vi "tm_getparameter_a.vi"(6 "Index":i32, 8 "error in (no error)":errorcluster, 10 "Parameter":u32(ring)=4215968 items=["SENSOR MODE"=4212128, "CCD MODE"=4212384, "READOUT MODE"=4211872, "ACTIVE VIEW INDEX"=4343136, "BITS PER CHANNEL"=4342976, "IMAGE PIXEL TYPE"=4343296, "BINNING"=4215968, "EXPOSURE TIME"=2049184, "CONTRAST GAIN"=3163312, "CONTRAST OFFSET"=3163328, "LIGHT MODE"=2114720, "SENSITIVITY"=2114992, "PHOTON IMAGING MODE"=2115200, "HIGH DYNAMIC RANGE MODE"=3163360, "WHITE BALANCE"=3163568, "TEMPERATURE"=2115232, "TEMPERATURE TARGET"=2115264, "SENSOR COOLER FAN"=2115296, "LINEBUNDLE HEIGHT"=4212192, "MECHANICAL SHUTTER"=2115488, "BACK FOCUS POSITION"=8422304, "TRIGGER CONNECTOR"=1066432, "TRIGGER SOURCE"=1066144, "OUTPUT TRIGGER SOURCE"=1852576, "TRIGGER GLOBAL EXPOSURE"=2049680, "FIRST TRIGGER BEHAVIOR"=2049696, "CHANNEL SYNC"=1852352, "READOUT DIRECTION"=4211904, "PRE HSYNC COUNT"=1852704, "INTERNAL LINE SPEED"=4191408, "INTERNAL LINE INTERVAL"=4191424], 11 "Handle in":u32) -> (0 "error out":errorcluster, 2 "Value out":dbl, 3 "Handle out":u32)   [LabVIEW 2015]
uses:
  tmcamcon.dll
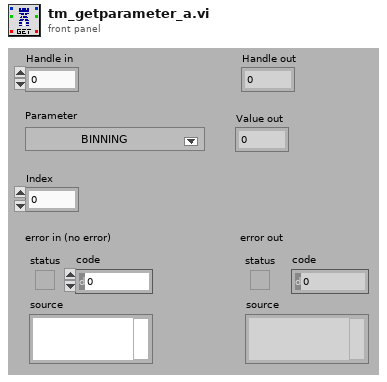
[diagram p1: front panel]
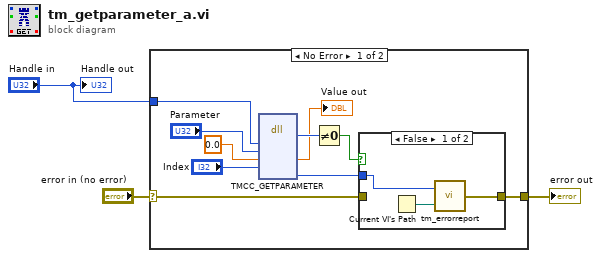
[diagram p0: block diagram]
diagram:
  n1 = case shown="No Error" "error in (no error)" {
    selector: "error in (no error)" -> [w8 w18]
    tunnel: [w5 w18] -> w2
    tunnel: "Handle in" -> [w12 _]
    frame No Error {
      n2 = dll-call lib="tmcamcon.dll" fn="TMCC_GETPARAMETER"("handle"=w12, "parameter"="Parameter", "value"=0.0, "view"="Index") -> ("return type"=w13:u32, "value"=→"Value out":dbl, "Erval"=w7:i32)  [unwired: 7 in, 2 out]
      n3 = Not Equal To 0?(x=w13) -> (x != 0?=w6:bool)
      n4 = case shown="False" w6 {
        tunnel: w8 -> [_ w17]
        tunnel: [w15 w17] -> w5
        tunnel: w7 -> [w14 _]
        frame False {
          n5 = Current VI's Path() -> (path=w16:path)
          n6 = call "tm_errorreport.vi"("Source"=w16, "Error"=w14) -> ("error out"=w15:errorcluster)
        }
        frame True {
        }
      }
    }
    frame Error {
    }
  }
  "error out" <- w2
  "Handle out" <- "Handle in"
